vi "Reset Hardware List and Run Button.vi"(8 "error in (no error)":errorcluster, 11 "Function UI in":refnum<class "Controller UI.lvclass">) -> (0 "error out":errorcluster, 3 "Function UI out":refnum<class "Controller UI.lvclass">)   [LabVIEW 2016, in "Controller UI.lvlib" / "Controller UI.lvclass"]
uses:
  <userlib>/Common Components/Controller UI/Controller UI.lvclass
  <userlib>/Common Components/Controller UI/Controller UI.lvclass/Controller UI.ctl
  <userlib>/Common Components/Controller UI/Accessors/Read Run.vi
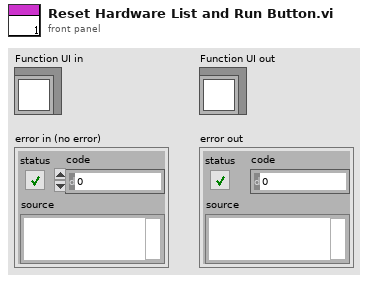
[diagram p1: front panel]
types:
  T1 = enum8{"Enabled", "Disabled", "Disabled and Grayed Out"}
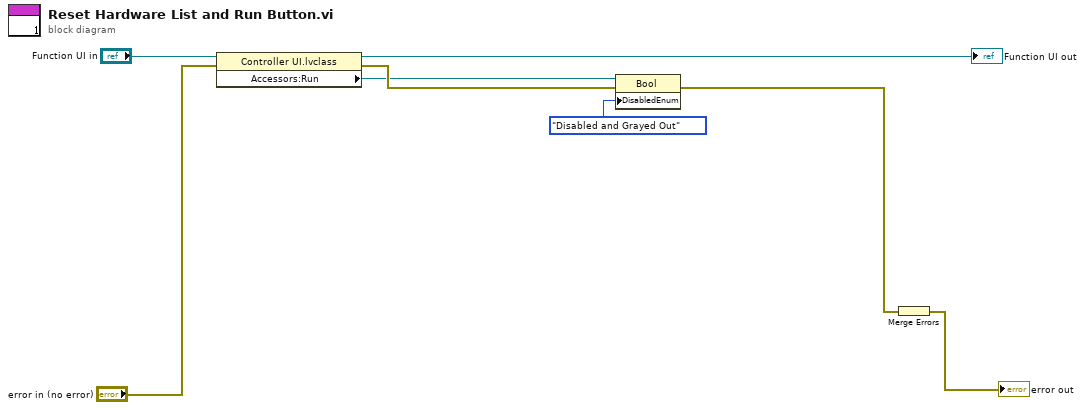
[diagram p0: block diagram]
diagram:
  n1 = property class="Controller UI.lvclass"(reference="Function UI in", error in="error in (no error)") -> (reference out=→"Function UI out":refnum<class "Controller UI.lvclass">, error out=w6:errorcluster, "Accessors:Run"=w5:refnum<vi>)
  n2 = property class="Bool"(reference=w5, error in=w6, "DisabledEnum"=T1."Disabled and Grayed Out" ("Disabled")) -> (error out=w7:errorcluster)  [unwired: 1 out]
  n3 = Merge Errors(w7) -> (→"error out":errorcluster)
